vi "Alternate Mark Inversion.vi"(6 "Phase In":dbl, 7 "Amplitude":dbl, 9 "Sampling Frequency":dbl=100000000.0, 10 "Frequency":dbl=1544000.0, 11 "Line Code":string) -> (1 "Samples Generated":i32, 2 "Signal":dbl[](array[numeric]), 3 "Time Axis":dbl[](array[numeric]), 4 "Phase Out":dbl)   [LabVIEW 2023]
doc: "Input phase of the signal"
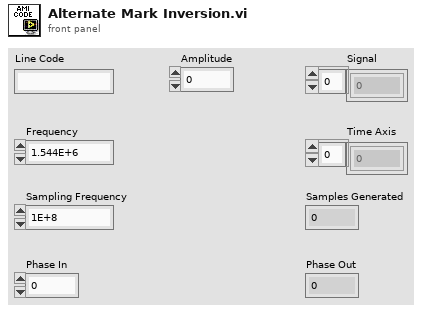
[diagram p1: front panel]
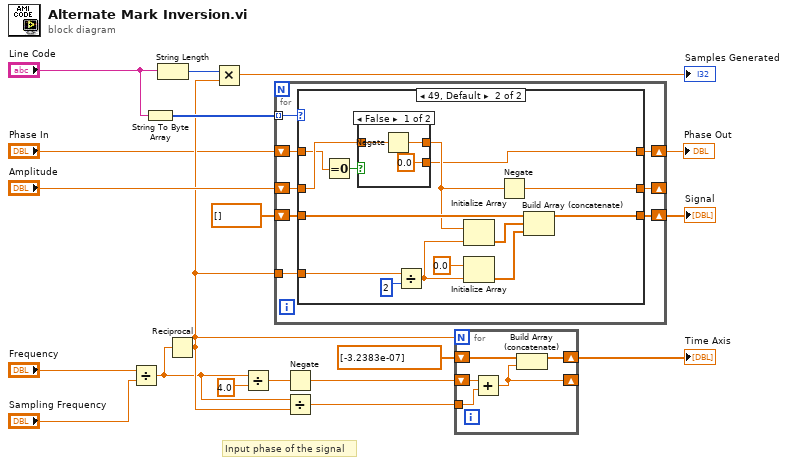
[diagram p0: block diagram]
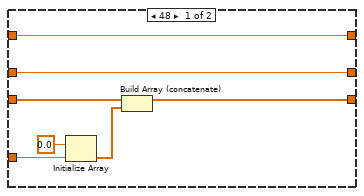
[diagram p2: hidden frame]
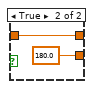
[diagram p3: hidden frame]
diagram:
  # "Input phase of the signal"
  n1 = Divide(x="Frequency", y="Sampling Frequency") -> (x/y=w5:dbl)
  n2 = String To Byte Array(string="Line Code") -> (unsigned byte array=w16:u8[])
  n3 = String Length(string="Line Code") -> (length=w19:i32)
  n4 = Reciprocal(x=w5) -> (1/x=w9:dbl)
  n5 = Multiply(x=w19, y=w9) -> (x*y=→"Samples Generated":dbl)
  n6 = Divide(x=w5, y=4.0) -> (x/y=w14:dbl)
  n7 = for {
    tunnel: w16 -> [w27] mode=indexing
    tunnel: w9 -> [w26]
    shift-right: [w25] -> w8
    shift-left: dbl[] [] -> [w24]
    shift-right: [w23] -> _
    shift-left: "Amplitude" -> [w22]
    shift-right: [w20] -> w1
    shift-left: "Phase In" -> [w21]
    n8 = case shown="49, Default" w27 {
      tunnel: w26 -> [w34 w48]
      tunnel: [w32 w45] -> w25
      tunnel: w24 -> [w31 w46]
      tunnel: [w29 w42] -> w23
      tunnel: w22 -> [w29 w40]
      tunnel: w21 -> [w28 w37]
      tunnel: [w28 w36] -> w20
      frame 48 {
        n9 = Initialize Array(0.0, w34) -> (w33:dbl[])
        n10 = Build Array (concatenate)(w31, w33) -> (w32:dbl[])
      }
      frame 49, Default {
        n11 = Equal To 0?(x=w37) -> (x = 0?=w41:bool)
        n12 = case shown="False" w41 {
          tunnel: [0.0 180.0] -> w36
          tunnel: w40 -> [w51 w53]
          tunnel: [w50 w53] -> w39
          frame False {
            n13 = Negate(x=w51) -> (-x=w50:dbl)
          }
          frame True {
          }
        }
        n14 = Divide(x=w48, y=2) -> (x/y=w47:dbl)
        n15 = Initialize Array(w39, w47) -> (w44:dbl[])
        n16 = Initialize Array(0.0, w47) -> (w43:dbl[])
        n17 = Negate(x=w39) -> (-x=w42:dbl)
        n18 = Build Array (concatenate)(w46, w44, w43) -> (w45:dbl[])
      }
    }
  }
  "Signal" <- w8
  "Phase Out" <- w1
  n19 = Negate(x=w14) -> (-x=w11:dbl)
  n20 = Divide(x=w5, y=w9) -> (x/y=w13:dbl)
  n21 = for {
    N: w9 -> [_]
    shift-right: [w54] -> _
    shift-left: w11 -> [w58]
    tunnel: w13 -> [w57]
    shift-right: [w55] -> w12
    shift-left: dbl[] [-3.2383e-07] -> [w56]
    n22 = Add(x=w58, y=w57) -> (x+y=w54:dbl)
    n23 = Build Array (concatenate)(w56, w54) -> (w55:dbl[])
  }
  "Time Axis" <- w12
